vi "SetpointSequence.vi"(2 "appended array":dbl[][](array[numeric]), 3 "Sweep rate (T/min)":dbl) -> (1 "Status":string)   [LabVIEW 2013]
uses:
  Exp VIs/global/B_Field_Global.vi
panel:
  out "Sections":i32 caption="of"
  out "Section":i32 caption="Running to vector"
  in  "Abort":bool
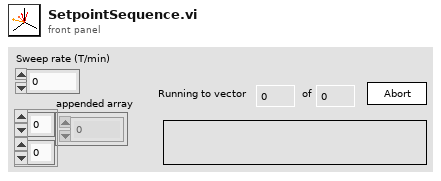
[diagram p1: front panel]
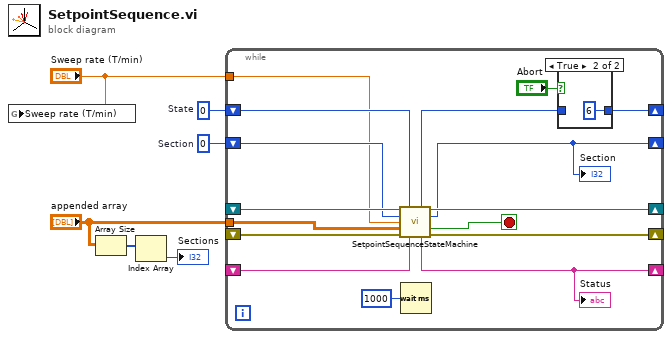
[diagram p0: block diagram]
diagram:
  w6 = 0  # Section
  w5 = 0  # State
  n1 = global write "B_Field_Global.vi" "Sweep rate (T/min)"("Sweep rate (T/min)") -> ()
  n2 = Array Size(array="appended array") -> (size(s)=w3:i32[])
  n3 = Index Array(array=w3) -> (element=→"Sections":i32)  [unwired: 1 in]
  n4 = while {
    shift-right: [w18] -> _
    shift-left: w5 -> [w16]
    shift-right: [w22] -> _
    shift-left: _ -> [w21]
    shift-right: [w19] -> _
    shift-left: _ -> [w20]
    tunnel: "appended array" -> [w14]
    shift-right: [w9] -> _
    shift-left: w6 -> [w15]
    shift-right: [w8] -> _
    shift-left: _ -> [w12]
    tunnel: "Sweep rate (T/min)" -> [w11]
    stop <- w13 stop-if-true
    n5 = call "SetpointSequenceStateMachine.vi"("VISA resource name in"=w21, "State in"=w16, "Section in"=w15, "Sweep rate"=w11, "Array of X,Y,Z setpoints"=w14, "error in"=w20, "Response in"=w12) -> ("State"=w17:i32, "VISA resource name out"=w22:refnum<visa-resource-name>, "Section"=w9:i32, "finished"=w13:bool, "Response"=w8:string, "error out"=w19:errorcluster)  [unwired: 3 in]
    "Section" <- w9
    "Status" <- w8
    n6 = Wait (ms)(milliseconds to wait=u32 1000) -> ()  [unwired: 1 out]
    n7 = case shown="True" "Abort" {
      tunnel: w17 -> [w23 _]
      tunnel: [w23 6] -> w18
      frame False {
      }
      frame True {
      }
    }
  }
